vi "Correct_Mistake_with_101-111_Connection-1.vi"(4 "error IN":errorcluster, 5 "[IN] # of Correc\nted Longest Track":i32, 6 "[IN] # of Prob\nlem Point Inside":i32, 7 "[IN] Still connected\ntracks in group":T2) -> (0 "error OUT":errorcluster, 3 "[OUT] Clusters for Re\nconstructed Tracks":T1)   [LabVIEW 2013]
doc: "Subprogram corrects the following mistake:\none of connected problem point misses the right status (instead of 111, 11 - 101, 1)"
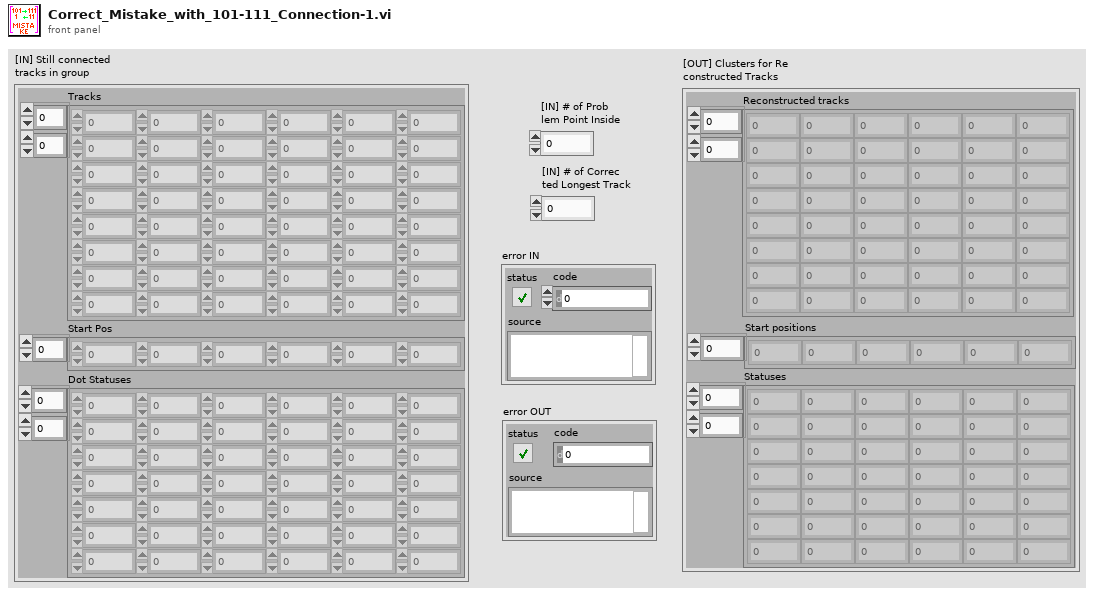
[diagram p1: front panel]
types:
  T1 = cluster{"Reconstructed tracks":dbl[][], "Start positions":i32[], "Statuses":i16[][]}
  T2 = cluster{"Tracks":dbl[][], "Start Pos":i32[], "Dot Statuses":i16[][]}
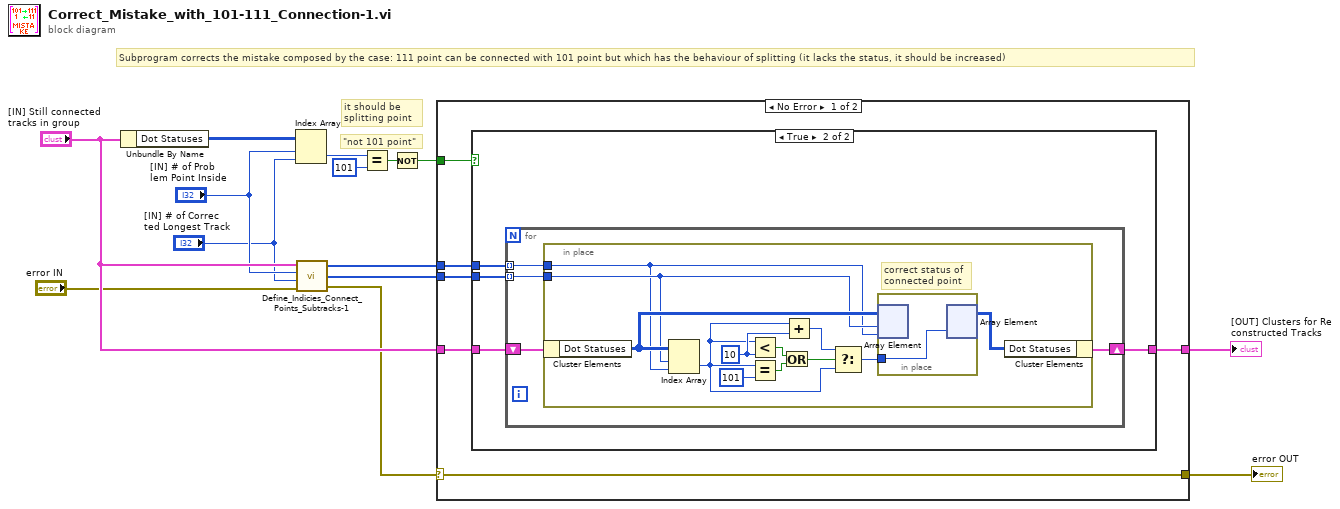
[diagram p0: block diagram]
diagram:
  # "it should be \nsplitting point"
  # "\"not 101 point\""
  # "Subprogram corrects the mistake composed by the case: 111 point can be connected with 101 point but which has the behaviour of splitting (it lacks the status, it should be increased)"
  n1 = Unbundle By Name("[IN] Still connected\ntracks in group") -> ("Dot Statuses"=w12:i16[][])
  n2 = Index Array(array=w12, index (row)="[IN] # of Prob\nlem Point Inside", index (col)="[IN] # of Correc\nted Longest Track") -> (element=w14:i16)
  n3 = call "Define_Indicies_Connect_Points_Subtracks-1.vi"("error IN"="error IN", "[IN] Index of track with\n(problem displacement)"="[IN] # of Correc\nted Longest Track", "[IN] Index of problem\ndisplacement inside track"="[IN] # of Prob\nlem Point Inside", "[IN] Track group"="[IN] Still connected\ntracks in group") -> ("error OUT"=w2:errorcluster, "[OUT] Index of \nconnected dots\ninside the track"=w3:i32[], "[OUT] Index of connected\ntracks with problem dot"=w4:i32[])
  n4 = Equal?(x=w14, y=i16 101) -> (x = y?=w11:bool)
  n5 = Not(x=w11) -> (.not. x?=w10:bool)
  n6 = case shown="No Error" w2 {
    selector: w2 -> [w15 w43]
    tunnel: w10 -> [w20 _]
    tunnel: w3 -> [w19 _]
    tunnel: w4 -> [w18 _]
    tunnel: "[IN] Still connected\ntracks in group" -> [w17 w44]
    tunnel: [w16 w44] -> w1
    tunnel: [w15 w43] -> w9
    frame No Error {
      n7 = case shown="True" w20 {
        tunnel: w19 -> [_ w24]
        tunnel: w18 -> [_ w25]
        tunnel: w17 -> [w21 w23]
        tunnel: [w21 w22] -> w16
        frame False {
        }
        frame True {
          n8 = for {
            tunnel: w25 -> [w28] mode=indexing
            tunnel: w24 -> [w27] mode=indexing
            shift-right: [w26] -> w22
            shift-left: w23 -> [w29]
            n9 = in-place {
              in-place-border: w28 -> [w30]
              in-place-border: w27 -> [w31]
              w38 = i16 10 ("y")
              # "correct status of \nconnected point"
              n10 = in-place-cluster #1(w29) -> ("Dot Statuses"=w35:i16[][])
              n11 = Index Array(array=w35, index (row)=w31, index (col)=w30) -> (element=w32:i16)
              n12 = Less?(x=w32, y=w38) -> (x < y?=w40:bool)
              n13 = Equal?(x=w32, y=i16 101) -> (x = y?=w39:bool)
              n14 = Or(x=w40, y=w39) -> (x .or. y?=w37:bool)
              n15 = Add(x=w32, y=w38) -> (x+y=w36:i16)
              n16 = Select(t=w36, s=w37, f=w32) -> (s? t:f=w33:i16)
              n17 = in-place {
                in-place-border: w33 -> [w42]
                n18 = in-place-array #2(w35, w31, w30) -> ()  [unwired: 1 out]
                n19 = in-place-array #2(w42) -> (w34:i16[][])  [unwired: 2 out]
              }
              n20 = in-place-cluster #1("Dot Statuses"=w34) -> (w26:T2)
            }
          }
        }
      }
    }
    frame Error {
    }
  }
  "[OUT] Clusters for Re\nconstructed Tracks" <- w1
  "error OUT" <- w9
